vi "Test Read DLL.vi"() -> ()   [LabVIEW 2020]
uses:
  C:/Users/dzoni/Documents/NJ/Playground/LV/TCP Client/client/builds/ClientApp1/ClientApp1.dll
  builds/ClientApp1/ClientApp1.dll
panel:
  out "ID":string
  out "Port":u16
  out "Data 2":string
  out "Data":string
  out "Address":string
  out "error out":errorcluster
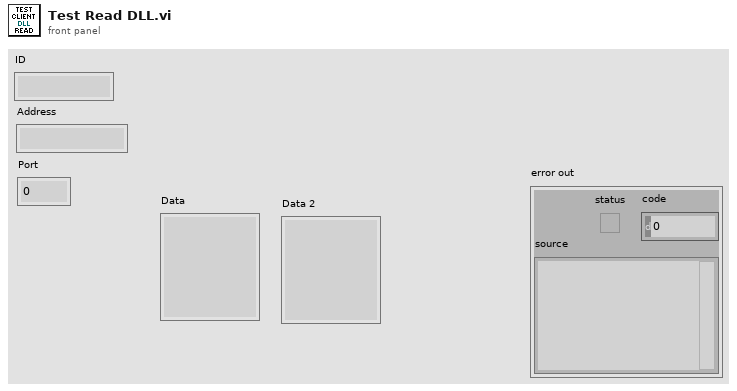
[diagram p1: front panel]
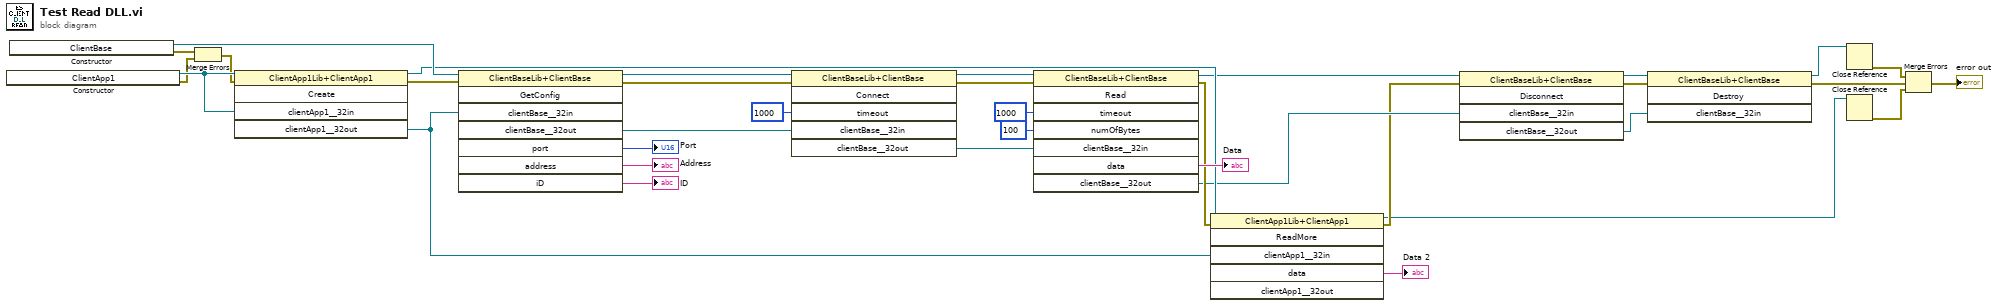
[diagram p0: block diagram]
diagram:
  n1 = constructor class="ClientApp1Lib+ClientApp1"() -> (reference out=w35:refnum<k24>, error out=w1:errorcluster)  [unwired: 3 in, 1 out]
  n2 = constructor class="ClientBaseLib+ClientBase"() -> (reference out=w34:refnum<k24>, error out=w3:errorcluster)  [unwired: 3 in, 1 out]
  n3 = Merge Errors(w3, w1) -> (w2:errorcluster)
  n4 = invoke class="ClientApp1Lib+ClientApp1" method="Create"(reference=w35, error in=w2, "clientApp1__32in"=w35) -> (reference out=w18:refnum<k24>, error out=w32:errorcluster, "clientApp1__32out"=w33:refnum<k24>)  [unwired: 2 in, 2 out]
  n5 = invoke class="ClientBaseLib+ClientBase" method="GetConfig"(reference=w34, error in=w32, "clientBase__32in"=w33) -> (reference out=w28:refnum<k24>, error out=w26:errorcluster, "clientBase__32out"=w27:refnum<k24>, "port"=→"Port":u16, "address"=→"Address":string, "iD"=→"ID":string)  [unwired: 5 in, 2 out]
  n6 = invoke class="ClientBaseLib+ClientBase" method="Connect"(reference=w28, error in=w26, "timeout"=1000, "clientBase__32in"=w27) -> (reference out=w24:refnum<k24>, error out=w23:errorcluster, "clientBase__32out"=w20:refnum<k24>)  [unwired: 2 in, 3 out]
  n7 = invoke class="ClientBaseLib+ClientBase" method="Read"(reference=w24, error in=w23, "timeout"=1000, "numOfBytes"=100, "clientBase__32in"=w20) -> (reference out=w14:refnum<k24>, error out=w17:errorcluster, "data"=→"Data":string, "clientBase__32out"=w15:refnum<k24>)  [unwired: 3 in, 4 out]
  n8 = invoke class="ClientApp1Lib+ClientApp1" method="ReadMore"(reference=w18, error in=w17, "clientApp1__32in"=w33) -> (reference out=w8:refnum<k24>, error out=w13:errorcluster, "data"=→"Data 2":string)  [unwired: 3 in, 3 out]
  n9 = invoke class="ClientBaseLib+ClientBase" method="Disconnect"(reference=w14, error in=w13, "clientBase__32in"=w15) -> (reference out=w10:refnum<k24>, error out=w11:errorcluster, "clientBase__32out"=w12:refnum<k24>)  [unwired: 2 in, 2 out]
  n10 = invoke class="ClientBaseLib+ClientBase" method="Destroy"(reference=w10, error in=w11, "clientBase__32in"=w12) -> (reference out=w9:refnum<k24>, error out=w7:errorcluster)  [unwired: 1 in, 2 out]
  n11 = Close Reference(reference=w9) -> (error out=w5:errorcluster)  [unwired: 1 in]
  n12 = Close Reference(reference=w8) -> (error out=w4:errorcluster)  [unwired: 1 in]
  n13 = Merge Errors(w5, w7, w4) -> (→"error out":errorcluster)
